vi "设置模块队列名.vi"() -> (2 "Msg":string)   [LabVIEW 2016, in "斯坦道CODcr.lvlib"]
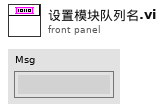
[diagram p1: front panel]
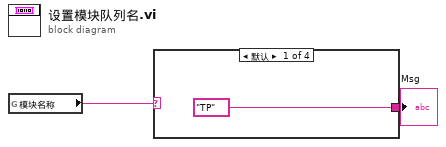
[diagram p0: block diagram]
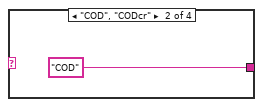
[diagram p2: hidden frame]
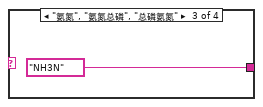
[diagram p3: hidden frame]
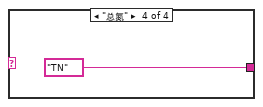
[diagram p4: hidden frame]
diagram:
  n1 = global read "VAR总磷总氮全局变量.vi" "模块名称"() -> (w1:string)
  n2 = case shown="默认" w1 {
    tunnel: ["TP" ("队列名") "COD" ("队列名") "NH3N" ("队列名") "TN" ("队列名")] -> w2
    frame Default {
    }
    frame "COD", "CODcr" {
    }
    frame "氨氮", "氨氮总磷", "总磷氨氮" {
    }
    frame "总氮" {
    }
  }
  "Msg" <- w2
